vi "practica12RNA.vi"() -> ()   [LabVIEW 2016]
panel:
  out "a 3":dbl
  in  "w 3":dbl[](array[numeric])
  in  "b 3":dbl
  in  "w 2":dbl[](array[numeric])
  in  "b 2":dbl
  out "a 2":dbl
  out "a":dbl
  in  "b":dbl
  in  "w":dbl[](array[numeric])
  in  "x":dbl[](array[numeric])
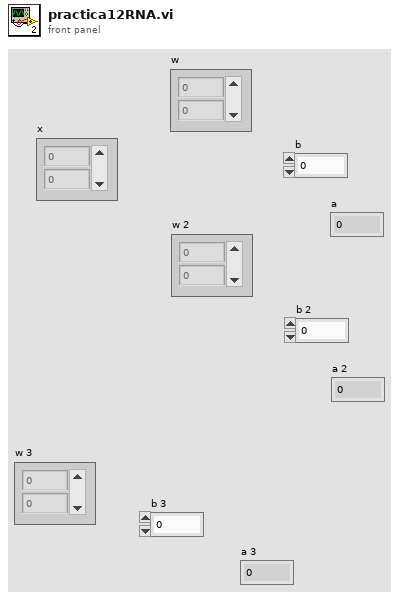
[diagram p1: front panel]
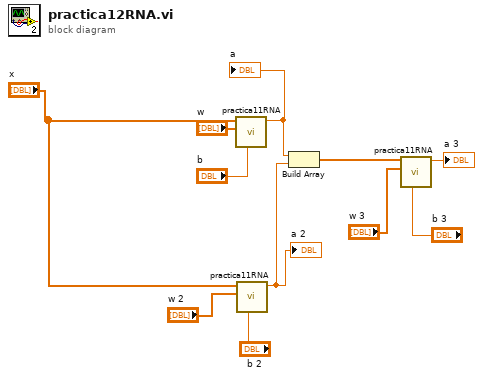
[diagram p0: block diagram]
diagram:
  n1 = call "practica11RNA.vi"("b"="b", "w"="w", "x"="x") -> ("a"=w5:dbl)  [unwired: 8 in]
  "a" <- w5
  n2 = call "practica11RNA.vi"("b"="b 2", "w"="w 2", "x"="x") -> ("a"=w4:dbl)  [unwired: 8 in]
  "a 2" <- w4
  n3 = Build Array(w5, w4) -> (w3:dbl[])
  n4 = call "practica11RNA.vi"("b"="b 3", "w"="w 3", "x"=w3) -> ("a"=→"a 3":dbl)  [unwired: 8 in]
